vi "Demo.vi"() -> ()   [LabVIEW 2023]
uses:
  C:/Mech-Mind/Mech-Eye SDK-2.5.0-c1-dev-01-17/API/dll/net48/MechEyeApiNet.dll
  dll/net48/MechEyeApiNet.dll
panel:
  in  "?":T1(tab)
  out "Color 2D Image":T2(plugin-control)
  out "Depth Map":T2(plugin-control)
  out "3D Point Cloud":refnum<vi>(3d-picture)
  in  "Parameter setting":enum32{"Connect & Capture", "Parameters"}(tab) caption="parameter"
  in  "Connect":bool
  in  "IP":string
  in  "Capture Once":bool
  in  "2D HDR Exposure Sequence":T3={"Exposure 1"=0.1, "Exposure 2"=0.1, "Exposure 3"=0.1, "Exposure 4"=0.1, "Exposure 5"=0.1} {"Exposure 5" min=0.1 max=999.0; "Exposure 4" min=0.1 max=999.0; "Exposure 3" min=0.1 max=999.0; "Exposure 2" min=0.1 max=999.0; "Exposure 1" min=0.1 max=999.0}
  in  "2D HDR Exposure Count":i32=1 min=1 max=5 step=1
  in  "2D Tone Mapping":bool
  in  "2D Auto-Exposure ROI":T4
  in  "2D Gray Value":i32=1 min=0 max=255 step=1
  in  "3D Exposure Sequence":T5={"Exposure 1"=0.1, "Exposure 2"=0.1, "Exposure 3"=0.1} {"Exposure 3" min=0.1 max=99.0; "Exposure 2" min=0.1 max=99.0; "Exposure 1" min=0.1 max=99.0}
  in  "3D Exposure Multiplier":i32=1 min=1 max=3 step=1
  in  "Stripe Contrast Threshold":i32 min=0 max=100 step=1
  in  "Point Cloud Outlier Removal":u8(ring) items=["Off", "Weak", "Normal", "Strong"]
  in  "Point Cloud Noise Removal":u8(ring) items=["Off", "Weak", "Normal", "Strong"]
  in  "Point Cloud Surface Smoothing":u8(ring) items=["Off", "Weak", "Normal", "Strong"]
  in  "ROI":T4
  in  "Depth Range":cluster{"lower":i32, "upper":i32}
  in  "3D Gain (0-16)":dbl
  in  "Set":bool
  in  "2D Exposure Time / ms":dbl=0.1 min=0.1 max=999.0
  in  "2D Exposure Mode":u16(ring) items=["Timed", "Auto", "HDR", "Flash"]
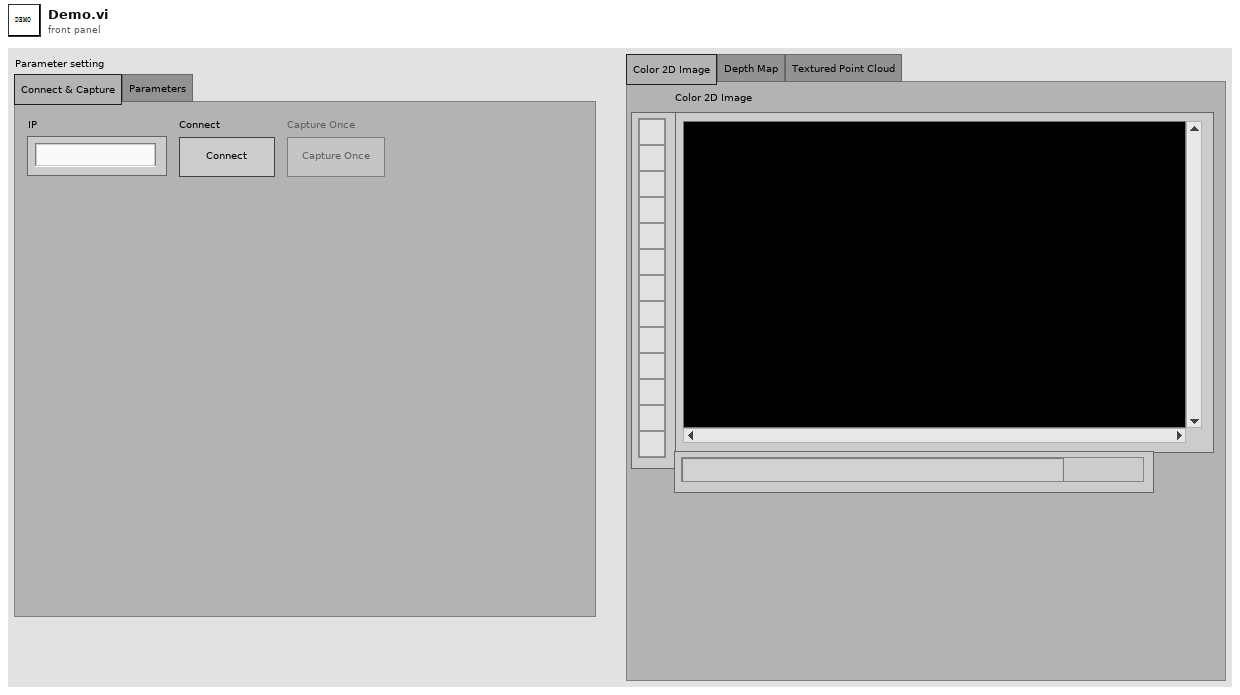
[diagram p1: front panel]
types:
  T1 = enum32{"Color 2D Image", "Depth Map", "Textured Point Cloud"}
  T2 = typedef "IMAQ Image.ctl" = refnum<image>
  T3 = cluster{"Exposure 1":dbl, "Exposure 2":dbl, "Exposure 3":dbl, "Exposure 4":dbl, "Exposure 5":dbl}
  T4 = cluster{"X":i32, "Y":i32, "Width":i32, "Height":i32}
  T5 = cluster{"Exposure 1":dbl, "Exposure 2":dbl, "Exposure 3":dbl}
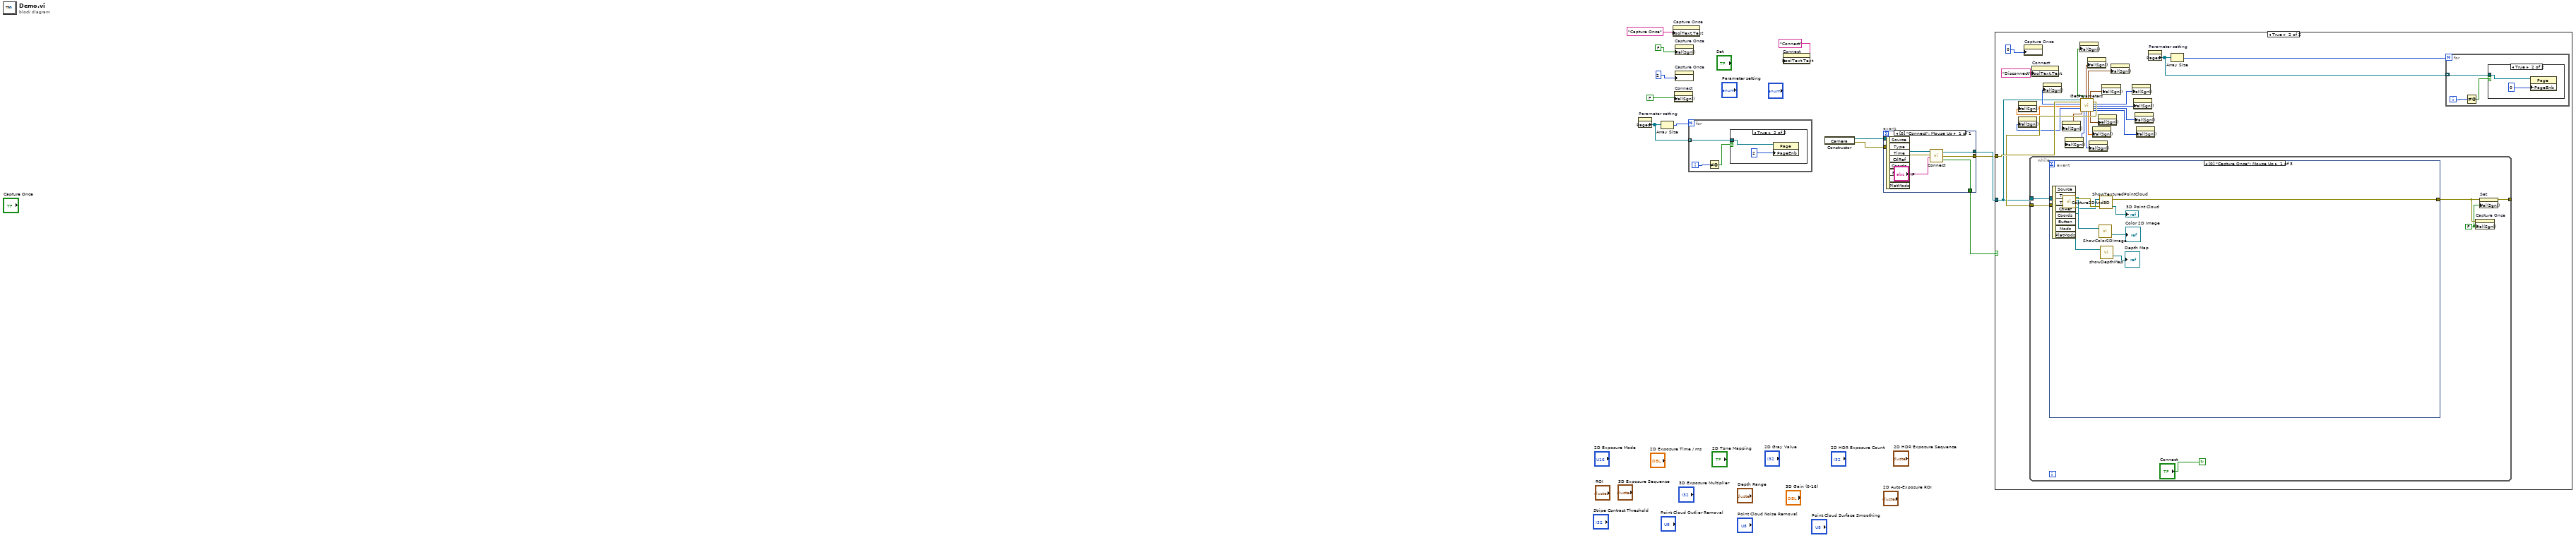
[diagram p0: block diagram]
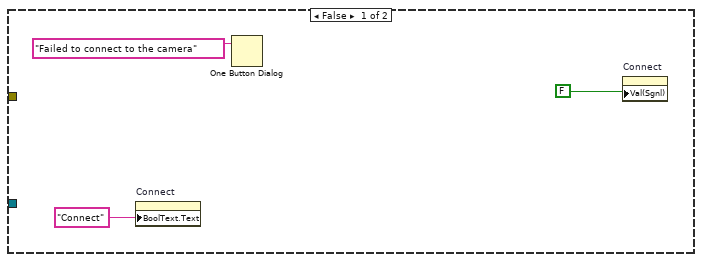
[diagram p3: hidden frame]
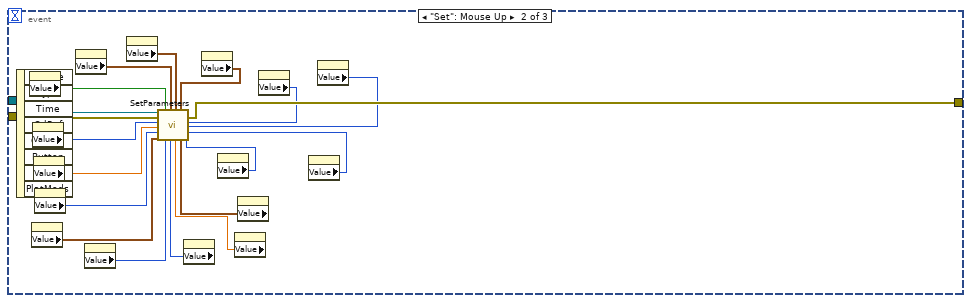
[diagram p5: hidden frame]
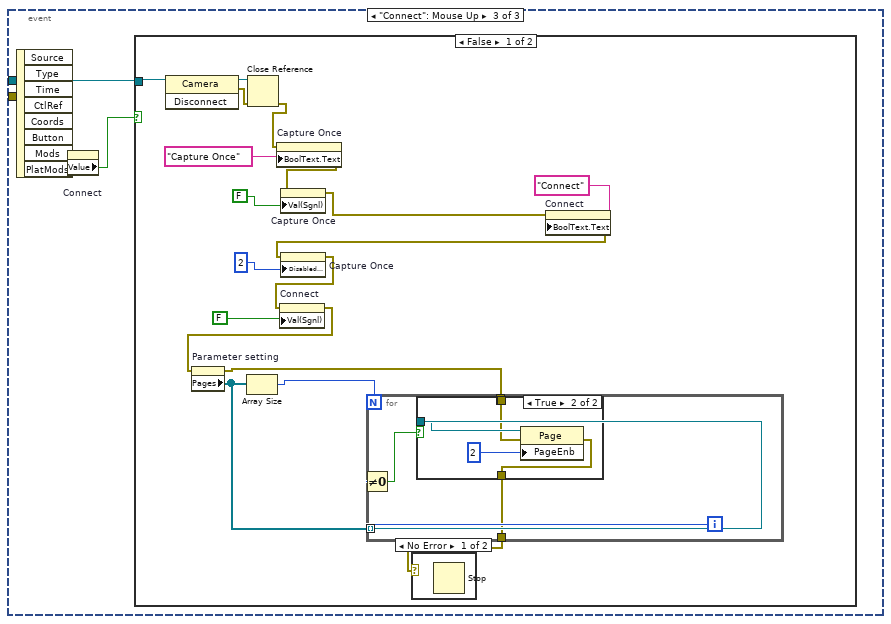
[diagram p6: hidden frame]
diagram:
  n1 = property on="Parameter setting" class="TabCtl (strict)"() -> ("Pages"=w2:refnum<vi>[])  [unwired: 2 in, 2 out]
  n2 = Array Size(array=w2) -> (size(s)=w3:i32)
  n3 = property on="Capture Once" class="Bool (strict)"("BoolText.Text"="Capture Once") -> ()  [unwired: 2 in, 2 out]
  n4 = property on="Connect" class="Bool (strict)"("Val(Sgnl)"=FALSE) -> ()  [unwired: 2 in, 2 out]
  n5 = property on="Capture Once" class="Bool (strict)"("Val(Sgnl)"=FALSE) -> ()  [unwired: 2 in, 2 out]
  n6 = property on="Capture Once" class="Bool (strict)"("DisabledEnum"=2) -> ()  [unwired: 2 in, 2 out]
  n7 = for {
    N: w3 -> [_]
    tunnel: w2 -> [w13] mode=indexing
    i -> [w15]
    n8 = Not Equal To 0?(x=w15) -> (x != 0?=w14:bool)
    n9 = case shown="True" w14 {
      tunnel: w13 -> [_ w17]
      frame False {
      }
      frame True {
        n10 = property class="Page"(reference=w17, "PageEnb"=2) -> ()  [unwired: 1 in, 2 out]
      }
    }
  }
  n11 = property on="Connect" class="Bool (strict)"("BoolText.Text"="Connect") -> ()  [unwired: 2 in, 2 out]
  n12 = constructor class="Camera"() -> (reference out=w7:refnum<k24>, error out=w12:errorcluster)  [unwired: 3 in, 1 out]
  n13 = event shown="[0] \"Connect\": Mouse Up" {
    selector: _ -> [_]
    dyn-events: _ -> [_]
    timeout: _ -> [_]
    tunnel: w7 -> [w23]
    tunnel: w12 -> [w22]
    tunnel: [w21] -> w6
    tunnel: [w20] -> w5
    tunnel: [w19] -> w4
    event "Connect": Mouse Up {
      n14 = event-data() -> ()  [unwired: 1 in, 8 out]
      n15 = call "Connect.vi"("IP Address"="IP", "error in (no error)"=w22, "MMind.Eye.Camera"=w23) -> ("Result"=w21:bool, "error out"=w19:errorcluster, "MMind.Eye.Camera"=w20:refnum<k24>)  [unwired: 1 in]
    }
  }
  n16 = case shown="True" w6 {
    tunnel: w5 -> [_ w27]
    tunnel: w4 -> [_ w45]
    frame False {
      n17 = property on="Connect" class="Bool (strict)"("BoolText.Text"="Connect") -> ()  [unwired: 2 in, 2 out]
      n18 = One Button Dialog(message="Failed to connect to the camera") -> ()  [unwired: 1 in, 1 out]
      n19 = property on="Connect" class="Bool (strict)"("Val(Sgnl)"=FALSE) -> ()  [unwired: 2 in, 2 out]
    }
    frame True {
      n20 = property on="Capture Once" class="Bool (strict)"("DisabledEnum"=0) -> ()  [unwired: 2 in, 2 out]
      n21 = property on="Connect" class="Bool (strict)"("BoolText.Text"="Disconnect") -> ()  [unwired: 2 in, 2 out]
      n22 = call "GetParameters.vi"("MMind.Eye.Camera"=w27, "error in (no error)"=w45) -> ("2D ExposureMode (Timed Auto HDR Flash)"=w43:enum16{"Timed", "Auto", "HDR", "Flash"}, "2D ExposureTime (0.1-999)"=w42:dbl, "2D Gray Value"=w41:i32, "2D Auto-Exposure ROI (x, y, width, height)"=w36:T4, "2D Tone Mapping"=w40:bool, "2D HDR Exposure Count"=w35:i32, "2D HDR Exposure Sequence"=w39:T3, "3D Exposure Multiplier"=w34:i32, "3D Exposure Sequence"=w38:T5, "3D Gain (0-16)"=w33:dbl, "Depth Range (lower upper)"=w37:cluster{"lower":i32, "upper":i32}, "ROI (x, y, width, height)"=w32:T4, "error out"=w44:errorcluster, "PointCloudSurfaceSmoothing (Off Weak Normal Strong)"=w31:u8, "PointCloudNoiseRemoval (Off Weak Normal Strong)"=w30:u8, "PointCloudOutlierRemoval (Off Weak Normal Strong)"=w29:u8, "Stripe Contrast Threshold (0-100)"=w28:i32)  [unwired: 1 out]
      n23 = property on="2D Gray Value" class="DigNum (strict)"("Val(Sgnl)"=w41) -> ()  [unwired: 2 in, 2 out]
      n24 = property on="2D Exposure Time / ms" class="DigNum (strict)"("Val(Sgnl)"=w42) -> ()  [unwired: 2 in, 2 out]
      n25 = while {
        tunnel: w27 -> [w59]
        tunnel: w44 -> [w60]
        tunnel: [w56] -> _
        stop <- "Connect" continue-if-true
        w57 = FALSE
        n26 = event shown="[0] \"Capture Once\": Mouse Up" {
          selector: _ -> [_ _ _]
          dyn-events: _ -> [_ _ _]
          timeout: _ -> [_ _ _]
          tunnel: w59 -> [w68 w89 w90]
          tunnel: w60 -> [w70 w88 _]
          tunnel: [w69 w87 _] -> w58
          event "Capture Once": Mouse Up {
            n27 = event-data() -> ()  [unwired: 1 in, 8 out]
            n28 = call "Capture2DAnd3D.vi"("error in (no error)"=w70, "MMind.Eye.Camera"=w68) -> ("MMind.Eye.TexturedPointCloud"=w64:refnum<k24>, "MMind.Eye.DepthMap"=w65:refnum<k24>, "error out"=w67:errorcluster, "MMind.Eye.Color2DImage"=w66:refnum<k24>)  [unwired: 3 out]
            n29 = call "ShowColor2DImage.vi"("MMind.Eye.Color2DImage"=w66) -> ("2D Image out"=→"Color 2D Image":T2)  [unwired: 1 in, 1 out]
            n30 = call "ShowTexturedPointCloud.vi"("error in (no error)"=w67, "MMind.Eye.TexturedPointCloud"=w64) -> ("SceneObject out"=→"3D Point Cloud":refnum<vi>, "error out"=w69:errorcluster)
            n31 = call "showDepthMap.vi"("MMind.Eye.DepthMap"=w65) -> ("2D Image out"=→"Depth Map":T2)  [unwired: 1 in, 1 out]
          }
          event "Set": Mouse Up {
            n32 = event-data() -> ()  [unwired: 1 in, 8 out]
            n33 = property on="2D Tone Mapping" class="Bool (strict)"() -> ("Value"=w77:bool)  [unwired: 2 in, 2 out]
            n34 = property on="2D Auto-Exposure ROI" class="Clust (strict)"() -> ("Value"=w83:T4)  [unwired: 2 in, 2 out]
            n35 = property on="2D Exposure Mode" class="Ring (strict)"() -> ("Value"=w86:u16)  [unwired: 2 in, 2 out]
            n36 = property on="2D Exposure Time / ms" class="DigNum (strict)"() -> ("Value"=w85:dbl)  [unwired: 2 in, 2 out]
            n37 = property on="2D Gray Value" class="DigNum (strict)"() -> ("Value"=w84:i32)  [unwired: 2 in, 2 out]
            n38 = property on="2D HDR Exposure Sequence" class="Clust (strict)"() -> ("Value"=w76:T3)  [unwired: 2 in, 2 out]
            n39 = property on="2D HDR Exposure Count" class="DigNum (strict)"() -> ("Value"=w82:i32)  [unwired: 2 in, 2 out]
            n40 = property on="3D Exposure Sequence" class="Clust (strict)"() -> ("Value"=w75:T5)  [unwired: 2 in, 2 out]
            n41 = property on="3D Exposure Multiplier" class="DigNum (strict)"() -> ("Value"=w81:i32)  [unwired: 2 in, 2 out]
            n42 = property on="Depth Range" class="Clust (strict)"() -> ("Value"=w74:cluster{"lower":i32, "upper":i32})  [unwired: 2 in, 2 out]
            n43 = property on="Stripe Contrast Threshold" class="DigNum (strict)"() -> ("Value"=w78:i32)  [unwired: 2 in, 2 out]
            n44 = property on="3D Gain (0-16)" class="DigNum (strict)"() -> ("Value"=w80:dbl)  [unwired: 2 in, 2 out]
            n45 = property on="ROI" class="Clust (strict)"() -> ("Value"=w79:T4)  [unwired: 2 in, 2 out]
            n46 = property on="Point Cloud Surface Smoothing" class="Ring (strict)"() -> ("Value"=w73:u8)  [unwired: 2 in, 2 out]
            n47 = property on="Point Cloud Outlier Removal" class="Ring (strict)"() -> ("Value"=w71:u8)  [unwired: 2 in, 2 out]
            n48 = property on="Point Cloud Noise Removal" class="Ring (strict)"() -> ("Value"=w72:u8)  [unwired: 2 in, 2 out]
            n49 = call "SetParameters.vi"("MMind.Eye.Camera"=w89, "error in (no error)"=w88, "2D Exposure Mode (Timed Auto HDR Flash)"=w86, "2D Exposure Time (0.1-999)"=w85, "2D Gray Value"=w84, "2D Auto-Exposure ROI (x, y, width, height)"=w83, "2D Tone Mapping"=w77, "2D HDR Exposure Count"=w82, "2D HDR Exposure Sequence"=w76, "3D Exposure Multiplier"=w81, "3D Exposure Sequence (value 0.1-99)"=w75, "3D Gain (0-16)"=w80, "Depth Range (lower upper)"=w74, "ROI (x, y, width, height)"=w79, "PointCloudSurfaceSmoothing (Off Weak Normal Strong)"=w73, "PointCloudNoiseRemoval (Off Weak Normal Strong)"=w72, "PointCloudOutlierRemoval (Off Weak Normal Strong)"=w71, "Stripe Contrast Thresold (0-100)"=w78) -> ("error out"=w87:errorcluster)  [unwired: 1 out]
          }
          event "Connect": Mouse Up {
            n50 = event-data() -> ()  [unwired: 1 in, 8 out]
            n51 = property on="Connect" class="Bool (strict)"() -> ("Value"=w91:bool)  [unwired: 2 in, 2 out]
            n52 = case shown="False" w91 {
              tunnel: w90 -> [w109 _]
              frame False {
                n53 = invoke class="Camera" method="Disconnect"(reference=w109) -> (reference out=w108:refnum<k24>, error out=w100:errorcluster)  [unwired: 2 in, 1 out]
                n54 = Close Reference(reference=w108, error in (no error)=w100) -> (error out=w99:errorcluster)
                n55 = property on="Capture Once" class="Bool (strict)"(error in=w99, "BoolText.Text"="Capture Once") -> (error out=w98:errorcluster)  [unwired: 1 in, 1 out]
                n56 = property on="Capture Once" class="Bool (strict)"(error in=w98, "Val(Sgnl)"=FALSE) -> (error out=w97:errorcluster)  [unwired: 1 in, 1 out]
                n57 = property on="Connect" class="Bool (strict)"(error in=w97, "BoolText.Text"="Connect") -> (error out=w96:errorcluster)  [unwired: 1 in, 1 out]
                n58 = property on="Capture Once" class="Bool (strict)"(error in=w96, "DisabledEnum"=2) -> (error out=w95:errorcluster)  [unwired: 1 in, 1 out]
                n59 = property on="Connect" class="Bool (strict)"(error in=w95, "Val(Sgnl)"=FALSE) -> (error out=w94:errorcluster)  [unwired: 1 in, 1 out]
                n60 = property on="Parameter setting" class="TabCtl (strict)"(error in=w94) -> (error out=w93:errorcluster, "Pages"=w102:refnum<vi>[])  [unwired: 1 in, 1 out]
                n61 = Array Size(array=w102) -> (size(s)=w103:i32)
                n62 = for {
                  N: w103 -> [_]
                  tunnel: w102 -> [w112] mode=indexing
                  tunnel: w93 -> [w110]
                  tunnel: [w111] -> w92
                  i -> [w114]
                  n63 = Not Equal To 0?(x=w114) -> (x != 0?=w113:bool)
                  n64 = case shown="True" w113 {
                    tunnel: w112 -> [_ w119]
                    tunnel: w110 -> [_ w117]
                    tunnel: [w115 w116] -> w111
                    tunnel: w110 -> [w115 _]
                    frame False {
                    }
                    frame True {
                      n65 = property class="Page"(reference=w119, error in=w117, "PageEnb"=2) -> (error out=w116:errorcluster)  [unwired: 1 out]
                    }
                  }
                }
                n66 = case shown="No Error" w92 {
                  frame No Error {
                    n67 = Stop() -> ()  [unwired: 1 in]
                  }
                  frame Error {
                  }
                }
              }
              frame True {
              }
            }
          }
        }
        n68 = property on="Capture Once" class="Bool (strict)"(error in=w58, "Val(Sgnl)"=w57) -> ()  [unwired: 1 in, 2 out]
        n69 = property on="Set" class="Bool (strict)"(error in=w58, "Val(Sgnl)"=w57) -> (error out=w56:errorcluster)  [unwired: 1 in, 1 out]
      }
      n70 = property on="2D Exposure Mode" class="Ring (strict)"("Val(Sgnl)"=w43) -> ()  [unwired: 2 in, 2 out]
      n71 = property on="2D Auto-Exposure ROI" class="Clust (strict)"("Val(Sgnl)"=w36) -> ()  [unwired: 2 in, 2 out]
      n72 = property on="2D HDR Exposure Count" class="DigNum (strict)"("Val(Sgnl)"=w35) -> ()  [unwired: 2 in, 2 out]
      n73 = property on="2D Tone Mapping" class="Bool (strict)"("Val(Sgnl)"=w40) -> ()  [unwired: 2 in, 2 out]
      n74 = property on="2D HDR Exposure Sequence" class="Clust (strict)"("Val(Sgnl)"=w39) -> ()  [unwired: 2 in, 2 out]
      n75 = property on="3D Exposure Multiplier" class="DigNum (strict)"("Val(Sgnl)"=w34) -> ()  [unwired: 2 in, 2 out]
      n76 = property on="3D Gain (0-16)" class="DigNum (strict)"("Val(Sgnl)"=w33) -> ()  [unwired: 2 in, 2 out]
      n77 = property on="ROI" class="Clust (strict)"("Val(Sgnl)"=w32) -> ()  [unwired: 2 in, 2 out]
      n78 = property on="Depth Range" class="Clust (strict)"("Val(Sgnl)"=w37) -> ()  [unwired: 2 in, 2 out]
      n79 = property on="3D Exposure Sequence" class="Clust (strict)"("Val(Sgnl)"=w38) -> ()  [unwired: 2 in, 2 out]
      n80 = property on="Point Cloud Surface Smoothing" class="Ring (strict)"("Val(Sgnl)"=w31) -> ()  [unwired: 2 in, 2 out]
      n81 = property on="Point Cloud Noise Removal" class="Ring (strict)"("Val(Sgnl)"=w30) -> ()  [unwired: 2 in, 2 out]
      n82 = property on="Point Cloud Outlier Removal" class="Ring (strict)"("Val(Sgnl)"=w29) -> ()  [unwired: 2 in, 2 out]
      n83 = property on="Stripe Contrast Threshold" class="DigNum (strict)"("Val(Sgnl)"=w28) -> ()  [unwired: 2 in, 2 out]
      n84 = property on="Parameter setting" class="TabCtl (strict)"() -> ("Pages"=w47:refnum<vi>[])  [unwired: 2 in, 2 out]
      n85 = Array Size(array=w47) -> (size(s)=w48:i32)
      n86 = for {
        N: w48 -> [_]
        tunnel: w47 -> [w50] mode=indexing
        i -> [w52]
        n87 = Not Equal To 0?(x=w52) -> (x != 0?=w51:bool)
        n88 = case shown="True" w51 {
          tunnel: w50 -> [_ w54]
          frame False {
          }
          frame True {
            n89 = property class="Page"(reference=w54, "PageEnb"=0) -> ()  [unwired: 1 in, 2 out]
          }
        }
      }
    }
  }
